vi "Plot.vi"(8 "error in":errorcluster, 11 "Plot Refnum":refnum<vi>) -> (0 "error out":errorcluster, 3 "Plot out":refnum<class "Plot.lvclass">)   [LabVIEW 2014, in "Plot.lvclass"]
uses:
  Plot.lvclass
  Plot.lvclass/Plot.ctl
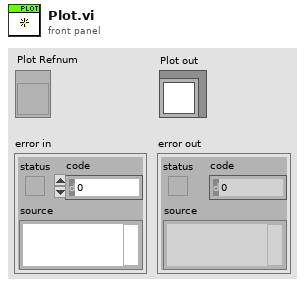
[diagram p1: front panel]
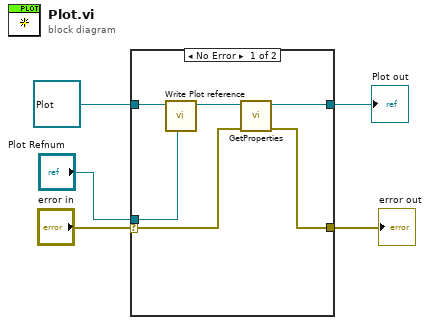
[diagram p0: block diagram]
diagram:
  n1 = case shown="No Error" "error in" {
    selector: "error in" -> [w6 w13]
    tunnel: "Plot Refnum" -> [w7 _]
    tunnel: refnum<class "Plot.lvclass"> refnum ("Scale in") -> [w9 w12]
    tunnel: [w10 w13] -> w3
    tunnel: [w11 w12] -> w4
    frame No Error {
      n2 = call "Write Plot reference.vi"("Plot reference"=w7, "Plot in"=w9) -> ("Plot out"=w8:refnum<class "Plot.lvclass">)  [unwired: 7 in]
      n3 = call-dynamic "GetProperties.vi"("error in"=w6, "Plot in"=w8) -> ("error out"=w10:errorcluster, "Plot out"=w11:refnum<class "Plot.lvclass">)  [unwired: 8 in]
    }
    frame Error {
    }
  }
  "error out" <- w3
  "Plot out" <- w4
